vi "Run Process.vi"(8 "error in (no error)":errorcluster, 11 "CoolApp in":refnum<class "CoolApp.lvclass">) -> (0 "error out":errorcluster, 3 "CoolApp out":refnum<class "CoolApp.lvclass">)   [LabVIEW 2020, in "LAF2024Q2.lvlib" / "CoolApp.lvclass"]
uses:
  CoolApp.lvclass
  C:/Program Files (x86)/National Instruments/LabVIEW 2020/vi.lib/ActorFramework/Actor/Actor.lvclass
  C:/dev/lv20CE/laf-2024-q2/LAF2024Q2/CoolAppProcess/CoolAppProcess.lvclass
  Process State.ctl
  <vilib>/ActorFramework/Actor/Actor.lvclass/Actor.ctl
  <vilib>/ActorFramework/Message Enqueuer/Message Enqueuer.lvclass/Message Enqueuer.ctl
  CoolApp.lvclass/CoolApp.ctl
  <vilib>/ActorFramework/Message Enqueuer/Init from Existing Queue.vi
  <vilib>/ActorFramework/Message Enqueuer/Enqueue.vi
  <vilib>/ActorFramework/Stop Msg/Stop Msg.lvclass
  C:/Program Files (x86)/National Instruments/LabVIEW 2020/vi.lib/ActorFramework/Message/Message.lvclass
  <vilib>/ActorFramework/Message Priority Queue/Priority Enqueue.vi
  <vilib>/ActorFramework/Message Enqueuer/Message Enqueuer.lvclass
  CoolAppProcess/CoolAppProcess.lvclass
  <vilib>/ActorFramework/Actor/Actor.lvclass
  LAF2024Q2.lvlib
panel:
  out "Log":string
  out "Chart":T1
  out "DAQ":T1
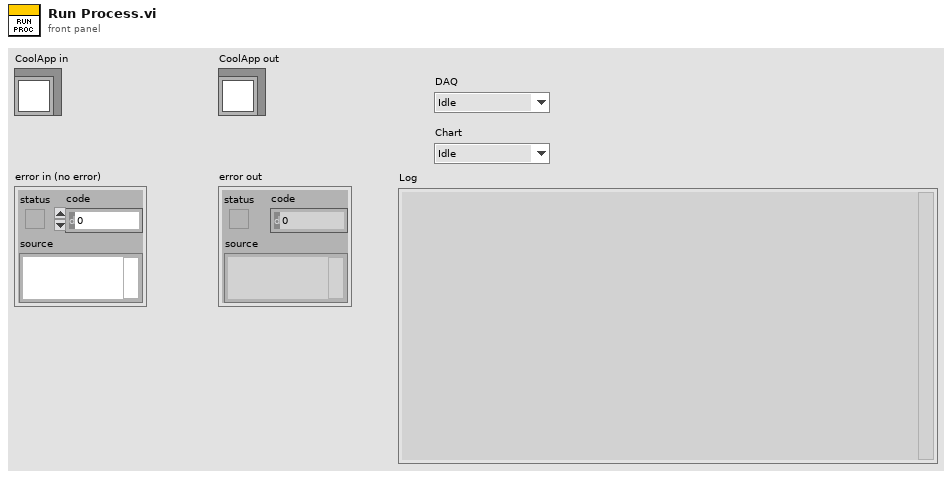
[diagram p1: front panel]
types:
  T1 = typedef "LAF2024Q2.lvlib/Process State.ctl" = enum16{"Idle", "Initializing", "Starting", "Running", "Stopping", "Stopped"}
  T2 = typedef "LAF2024Q2.lvlib/CoolApp.lvclass/Nested.ctl" = enum16{"DAQ", "Chart"}
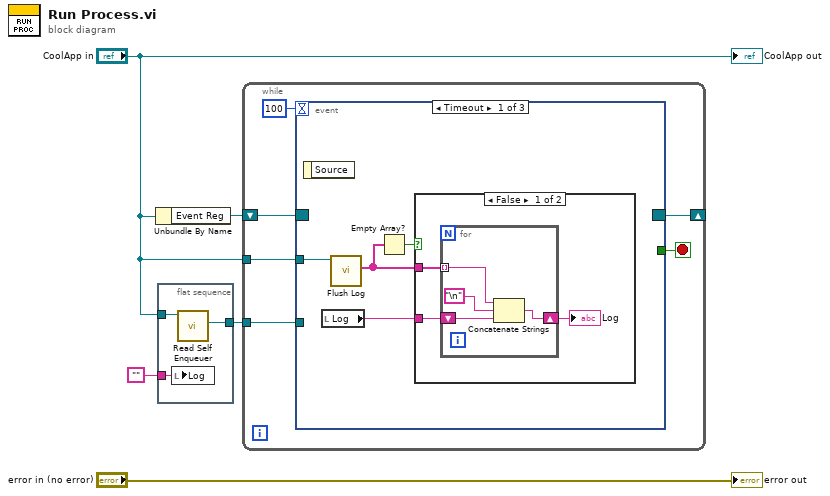
[diagram p0: block diagram]
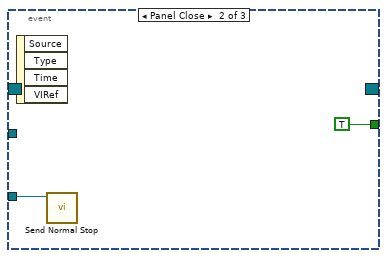
[diagram p3: hidden frame]
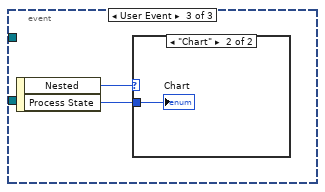
[diagram p4: hidden frame]
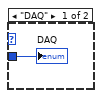
[diagram p5: hidden frame]
diagram:
  n1 = Unbundle By Name("CoolApp in") -> ("Event Reg"=w4:refnum<event-registration>)
  n2 = flat-sequence {
    tunnel: "CoolApp in" -> [w8]
    tunnel: [w7] -> w2
    tunnel: "" -> [w6]
    frame #0 {
      n3 = local write "Log"(w6) -> ()
      n4 = call <vilib>:"Read Self Enqueuer.vi"("Actor"=w8) -> ("Self Enqueuer"=w7:refnum<class "Message Enqueuer.lvclass">)  [unwired: 10 in]
    }
  }
  n5 = while {
    shift-right: [w13] -> _
    shift-left: w4 -> [w14]
    tunnel: "CoolApp in" -> [w11]
    tunnel: w2 -> [w10]
    stop <- w9 stop-if-true
    n6 = event shown="[0] Timeout" {
      selector: w14 -> [_ _ _]
      dyn-events: [_ _ _] -> w13
      timeout: 100 -> [_ _ _]
      tunnel: w11 -> [w18 _ _]
      tunnel: w10 -> [_ w26 _]
      tunnel: [_ TRUE _] -> w9
      event Timeout {
        n7 = event-data() -> ()  [unwired: 1 in, 1 out]
        n8 = local read "Log"() -> (w17:string)
        n9 = call "Flush Log.vi"("CoolAppProcess in"=w18) -> ("remaining elements"=w16:string[])  [unwired: 8 in, 2 out]
        n10 = Empty Array?(array=w16) -> (empty?=w15:bool)
        n11 = case shown="False" w15 {
          tunnel: w17 -> [w21 _]
          tunnel: w16 -> [w19 _]
          frame False {
            n12 = for {
              shift-right: [w24] -> w20
              shift-left: w21 -> [w25]
              tunnel: w19 -> [w22] mode=indexing
              n13 = Concatenate Strings(w22, "\n", w25) -> (w24:string)
            }
            "Log" <- w20
          }
          frame True {
          }
        }
      }
      event Panel Close {
        n14 = event-data() -> ()  [unwired: 1 in, 4 out]
        n15 = call <vilib>:"Send Normal Stop.vi"("Message Enqueuer"=w26) -> ()  [unwired: 10 in, 1 out]
      }
      event User Event {
        n16 = event-data() -> ("Nested"=w29:T2, "Process State"=w28:T1)  [unwired: 1 in]
        n17 = case shown="\"Chart\"" w29 {
          tunnel: w28 -> [w30 w31]
          frame "DAQ" {
            "DAQ" <- w30
          }
          frame "Chart" {
            "Chart" <- w31
          }
        }
      }
    }
  }
  "error out" <- "error in (no error)"
  "CoolApp out" <- "CoolApp in"
